vi "Query Lock In Amplifier Status.vi"(8 "error in (no error)":errorcluster, 11 "VISA resource name":refnum<visa-resource-name>) -> (0 "error out":errorcluster, 2 "Lock In Amplifier Data Message":string, 3 "VISA resource name out":refnum<visa-resource-name>)   [LabVIEW 2020, in "Stanford Research SR865.lvlib"]
doc: "Queries the Lock-In Amplifier Status register for the Questionable Data Register group. Essentially, it is used to observe possible invalid results. s"
uses:
  Stanford Research SR865.lvlib
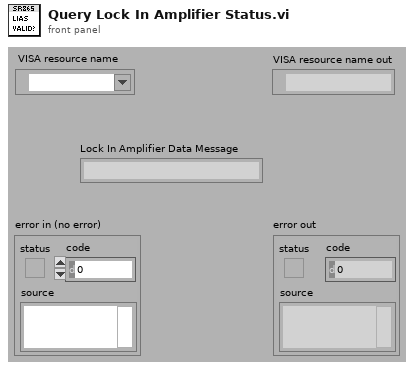
[diagram p1: front panel]
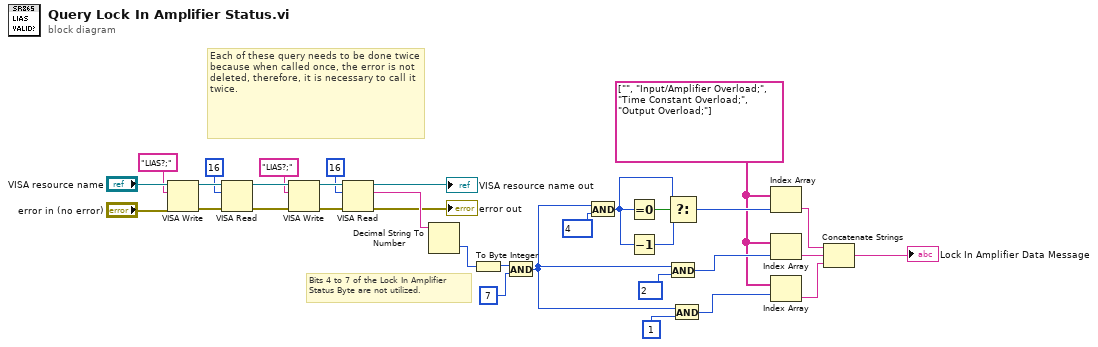
[diagram p0: block diagram]
diagram:
  w10 = string[] ["", "Input/Amplifier Overload;", "Time Constant Overload;", "Output Overload;"]
  # "Each of these query needs to be done twice because when called once, the error is not deleted, therefore, it is necessary to call it twice."
  # "Bits 4 to 7 of the Lock In Amplifier Status Byte are not utilized."
  n1 = VISA Write(VISA resource name="VISA resource name", write buffer="LIAS?;", error in (no error)="error in (no error)") -> (VISA resource name out=w5:refnum<visa-resource-name>, error out=w6:errorcluster)  [unwired: 1 out]
  n2 = VISA Read(VISA resource name=w5, byte count=u32 16, error in (no error)=w6) -> (VISA resource name out=w29:refnum<visa-resource-name>, error out=w30:errorcluster)  [unwired: 2 out]
  n3 = VISA Write(VISA resource name=w29, write buffer="LIAS?;", error in (no error)=w30) -> (VISA resource name out=w27:refnum<visa-resource-name>, error out=w28:errorcluster)  [unwired: 1 out]
  n4 = VISA Read(VISA resource name=w27, byte count=u32 16, error in (no error)=w28) -> (VISA resource name out=→"VISA resource name out":refnum<visa-resource-name>, read buffer=w33:string, error out=→"error out":errorcluster)  [unwired: 1 out]
  n5 = Decimal String To Number(string=w33) -> (number=w2:i32)  [unwired: 2 in, 1 out]
  n6 = To Byte Integer(number=w2) -> (8bit integer=w11:i8)
  n7 = And(x=w11, y=i8 7 ("value")) -> (x .and. y?=w24:i8)
  n8 = And(x=w24, y=i8 4) -> (x .and. y?=w21:i8)
  n9 = Equal To 0?(x=w21) -> (x = 0?=w16:bool)
  n10 = Decrement(x=w21) -> (x-1=w17:i8)
  n11 = Select(t=w21, s=w16, f=w17) -> (s? t:f=w18:i8)
  n12 = And(x=w24, y=i8 2) -> (x .and. y?=w19:i8)
  n13 = And(x=w24, y=i8 1) -> (x .and. y?=w20:i8)
  n14 = Index Array(array=w10, index=w18) -> (element=w15:string)
  n15 = Index Array(array=w10, index=w19) -> (element=w22:string)
  n16 = Index Array(array=w10, index=w20) -> (element=w23:string)
  n17 = Concatenate Strings(w15, w22, w23) -> (→"Lock In Amplifier Data Message":string)
